vi "Name Value Sort for New.vi"(7 "Organized Name Values":string[][](array[string])) -> (8 "Sorted":string[][](array[string]))   [LabVIEW 2020]
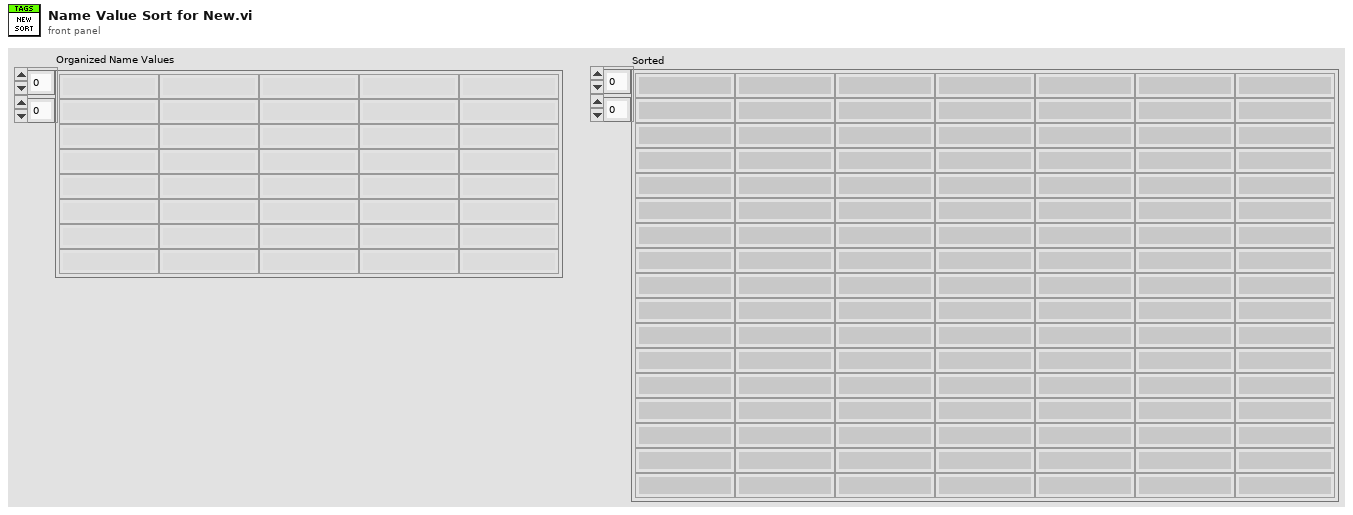
[diagram p1: front panel]
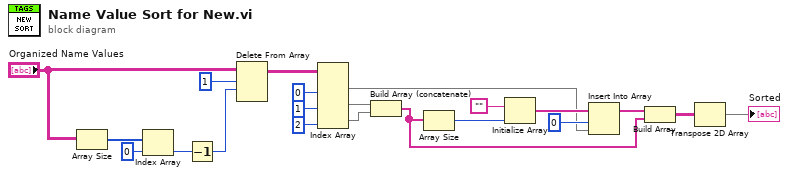
[diagram p0: block diagram]
diagram:
  n1 = Array Size(array="Organized Name Values") -> (size(s)=w9:i32[])
  n2 = Index Array(array=w9, index=0) -> (element=w7:i32)
  n3 = Decrement(x=w7) -> (x-1=w4:i32)
  n4 = Delete From Array(array="Organized Name Values", length=1, index (row)=w4) -> (array with subset deleted=w3:string[][])  [unwired: 1 in, 1 out]
  n5 = Index Array(array=w3, index (col) #1=0 ("disabled index (col)"), index (col) #2=1 ("index (col)"), index (col) #3=2 ("index (col)")) -> (element #1=w12:string[], element #2=w18:string[], element #3=w17:string[])  [unwired: 3 in]
  n6 = Build Array (concatenate)(w18, w17) -> (w10:string[])
  n7 = Array Size(array=w10) -> (size(s)=w16:i32)
  n8 = Initialize Array("", w16) -> (w14:string[])
  n9 = Insert Into Array(array=w14, index=0, new element=w12) -> (w11:string[])
  n10 = Build Array(w11, w10) -> (w2:string[][])
  n11 = Transpose 2D Array(2D array=w2) -> (transposed array=→"Sorted":string[][])
